vi "Model Initial Values - Fast Get Model Data.vi"(8 "error in (no error)":errorcluster, 11 "Local Model Ref in":T1 format="%.0x") -> (0 "error out":errorcluster, 1 "Inport Default Values":dbl[](array[numeric]), 2 "Inport Names":string[](array[string]), 3 "Local Model Ref out":T1 format="%.0x", 4 "Num Inports":i32, 5 "Inport Refs":T1[](array[typedef]) format="%.0x")   [LabVIEW 2011, in "Model Initial Values Custom Device.lvlib"]
uses:
  Model Initial Values Custom Device.lvlib
  <vilib>/NI Veristand/Custom Device API/Custom Device Item Ref.ctl
  Model Initial Values - Global.vi
  <vilib>/NI Veristand/Custom Device API/Get Item Property (Dependent Node Pointer).vi
  <vilib>/NI Veristand/Custom Device API/Get Item Property (String).vi
  <vilib>/NI Veristand/Custom Device API/Set Item Property (String).vi
  <vilib>/NI Veristand/Custom Device API/Set Item Property (String Array).vi
  <vilib>/NI Veristand/Custom Device API/Set Item Property (Double Array).vi
  <vilib>/NI Veristand/Custom Device API/Set Item Property (I32).vi
  <vilib>/NI Veristand/Custom Device API/Get Item Property (String Array).vi
  <vilib>/NI Veristand/Custom Device API/Get Item Property (Double Array).vi
  <vilib>/NI Veristand/Custom Device API/Get Item Property (I32).vi
  <vilib>/NI Veristand/Custom Device API/Custom Device API.lvlib
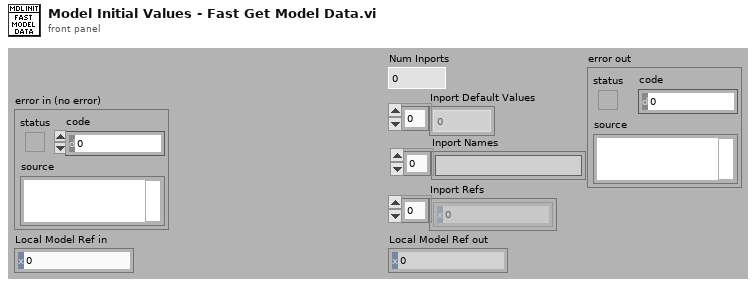
[diagram p1: front panel]
types:
  T1 = typedef "Custom Device API.lvlib/Custom Device Item Ref.ctl" = u64
  T2 = cluster{"Name":string, "Is Channel":bool, "GUID":string}
  T3 = cluster{"DLLSize":i32, "Timestamp":dbl, "MD5":string}
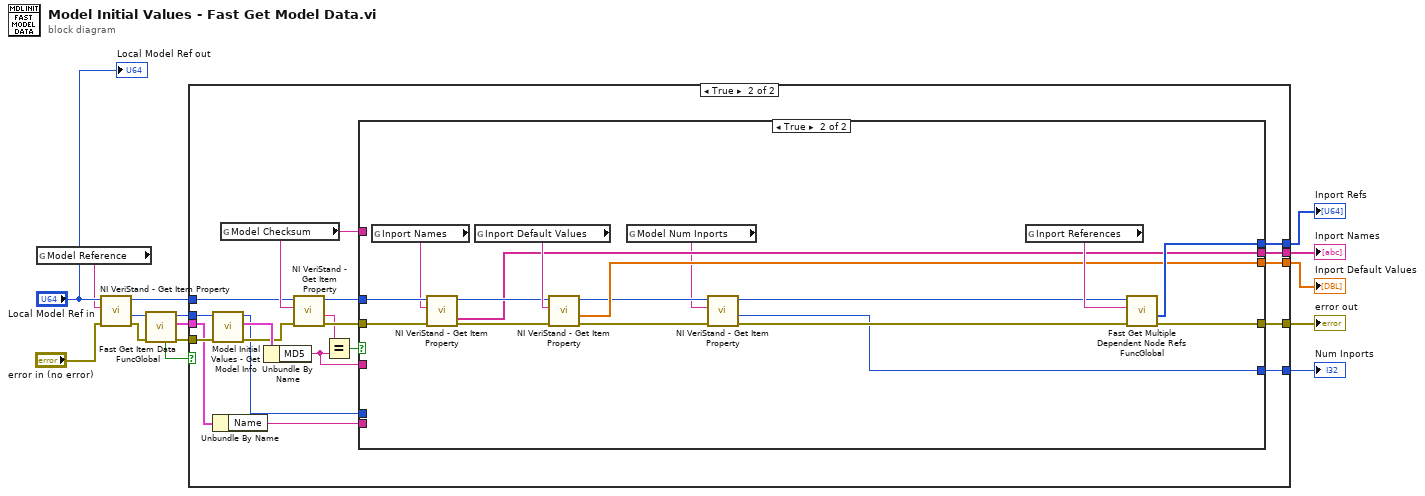
[diagram p0: block diagram]
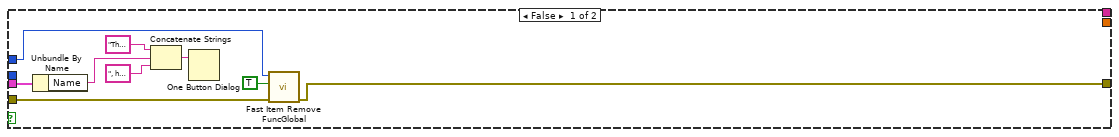
[diagram p2: hidden frame]
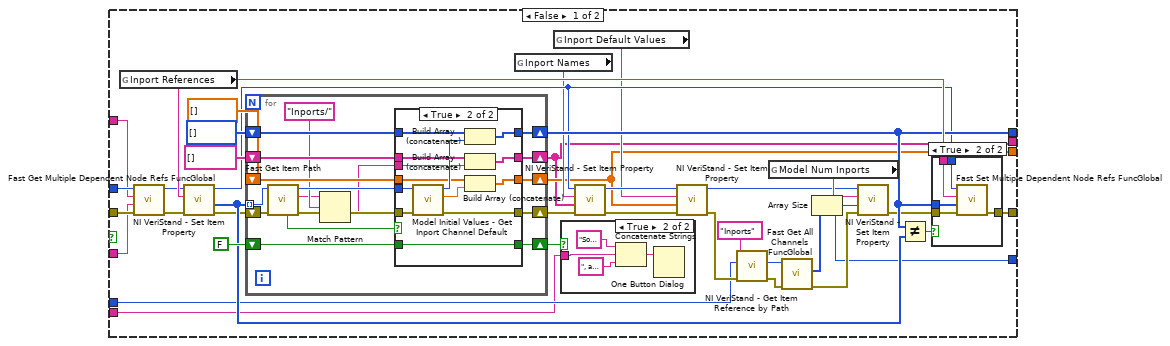
[diagram p3: hidden frame]
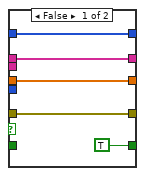
[diagram p6: hidden frame]
diagram:
  n1 = global read "Model Initial Values - Global.vi" "Model Reference"() -> (w12:string)
  n2 = call-poly <vilib>:"NI VeriStand - Get Item Property.vi"("error in (no error)"="error in (no error)", "Property Name"=w12, "Item Ref in"="Local Model Ref in") -> ("error out"=w6:errorcluster, "Dependent Node Ref"=w4:T1, "Item Ref out"=w14:T1)  [unwired: 5 in, 1 out]
  n3 = call "Fast Get Item Data FuncGlobal.vi"("error in (no error)"=w6, "Item Ref in"=w4) -> ("error out"=w5:errorcluster, "Item Info"=w2:T2, "Item Ref out"=w3:T1, "Found"=w1:bool)  [unwired: 6 in]
  n4 = case shown="True" w1 {
    tunnel: w14 -> [w17 w35]
    tunnel: [_ w33] -> w11
    tunnel: [_ w32] -> w10
    tunnel: [_ w31] -> w9
    tunnel: [_ w30] -> w8
    tunnel: [w16 w29] -> w7
    tunnel: w5 -> [w18 w28]
    tunnel: w3 -> [_ w27]
    tunnel: w2 -> [w24 w26]
    frame False {
      n5 = Unbundle By Name(w24) -> ("Name"=w19:string)
      n6 = Concatenate Strings("The model, " ("message"), w19, ", has been deleted from the project and will therefore be removed from this custom device." ("message")) -> (w22:string)
      n7 = One Button Dialog(message=w22) -> ()  [unwired: 1 in, 1 out]
      n8 = call "Fast Item Remove FuncGlobal.vi"("error in (no error)"=w18, "Force Delete (F)"=TRUE, "Item Ref in"=w17) -> ("error out"=w16:errorcluster)  [unwired: 7 in, 1 out]
    }
    frame True {
      n9 = call "Model Initial Values - Get Model Info.vi"("error in (no error)"=w28, "ID in"=w27) -> ("error out"=w42:errorcluster, "output cluster"=w43:T3, "ID out"=w34:T1)  [unwired: 7 in]
      n10 = Unbundle By Name(w26) -> ("Name"=w25:string)
      n11 = global read "Model Initial Values - Global.vi" "Model Checksum"() -> (w37:string)
      n12 = Unbundle By Name(w43) -> ("MD5"=w36:string)
      n13 = call-poly <vilib>:"NI VeriStand - Get Item Property.vi"("error in (no error)"=w42, "Property Name"=w37, "Item Ref in"=w35) -> ("error out"=w40:errorcluster, "Value"=w39:string, "Item Ref out"=w41:T1)  [unwired: 5 in, 1 out]
      n14 = Equal?(x=w39, y=w36) -> (x = y?=w38:bool)
      n15 = case shown="True" w38 {
        tunnel: [w76 w136] -> w29
        tunnel: w41 -> [w60 w141]
        tunnel: [w72 w134] -> w30
        tunnel: w40 -> [w63 w142]
        tunnel: w37 -> [w59 _]
        tunnel: w36 -> [w58 _]
        tunnel: [w57 w132] -> w32
        tunnel: [w56 w133] -> w31
        tunnel: [w45 w126] -> w33
        tunnel: w34 -> [w54 _]
        tunnel: w25 -> [w44 _]
        frame False {
          n16 = global read "Model Initial Values - Global.vi" "Inport References"() -> (w74:string)
          n17 = call-poly <vilib>:"NI VeriStand - Set Item Property.vi"("error in (no error)"=w63, "Value"=w58, "Property Name"=w59, "Item Ref in"=w60) -> ("error out"=w62:errorcluster, "Item Ref out"=w61:T1)  [unwired: 5 in, 1 out]
          n18 = call "Fast Get Multiple Dependent Node Refs FuncGlobal.vi"("error in (no error)"=w62, "Base Property Name"=w74, "Item Ref in"=w61) -> ("error out"=w71:errorcluster, "Dependent Node Refs"=w73:T1[], "Item Ref out"=w68:T1)  [unwired: 6 in]
          n19 = for {
            tunnel: w73 -> [w96] mode=indexing
            shift-right: [w106] -> w69
            shift-left: w71 -> [w100]
            shift-right: [w107] -> w56
            shift-left: string[] [] -> [w105]
            shift-right: [w103] -> w72
            shift-left: T1[] [] -> [w104]
            shift-right: [w102] -> w77
            shift-left: FALSE -> [w101]
            shift-right: [w94] -> w57
            shift-left: dbl[] [] -> [w95]
            n20 = call "Fast Get Item Path.vi"("error in (no error)"=w100, "Item Ref in"=w96) -> ("error out"=w99:errorcluster, "Path"=w92:string, "Item Ref out"=w97:T1, "Found"=w98:bool)  [unwired: 6 in]
            n21 = Match Pattern(string=w92, regular expression="Inports/") -> (after substring=w91:string)  [unwired: 1 in, 3 out]
            n22 = case shown="True" w98 {
              tunnel: [w111 w122] -> w107
              tunnel: w91 -> [_ w116]
              tunnel: w97 -> [_ w125]
              tunnel: w99 -> [w110 w124]
              tunnel: [w110 w123] -> w106
              tunnel: w105 -> [w111 w121]
              tunnel: w104 -> [w112 w119]
              tunnel: [w112 w118] -> w103
              tunnel: [TRUE w117] -> w102
              tunnel: w101 -> [_ w117]
              tunnel: w95 -> [w108 w114]
              tunnel: [w108 w113] -> w94
              frame False {
              }
              frame True {
                n23 = call "Model Initial Values - Get Inport Channel Default.vi"("error in"=w124, "Item Ref in"=w125) -> ("error out"=w123:errorcluster, "Default Value"=w115:dbl, "Item Ref out"=w120:T1)  [unwired: 6 in]
                n24 = Build Array (concatenate)(w119, w120) -> (w118:T1[])
                n25 = Build Array (concatenate)(w121, w116) -> (w122:string[])
                n26 = Build Array (concatenate)(w114, w115) -> (w113:dbl[])
              }
            }
          }
          n27 = global read "Model Initial Values - Global.vi" "Inport Names"() -> (w67:string)
          n28 = global read "Model Initial Values - Global.vi" "Inport Default Values"() -> (w64:string)
          n29 = case shown="True" w77 {
            tunnel: w44 -> [_ w87]
            frame False {
            }
            frame True {
              n30 = Concatenate Strings("Some inports have been deleted from the model, " ("message"), w87, ", and will therefore be removed from the \"Model Initial Values\" custom device." ("message")) -> (w88:string)
              n31 = One Button Dialog(message=w88) -> ()  [unwired: 1 in, 1 out]
            }
          }
          n32 = call-poly <vilib>:"NI VeriStand - Set Item Property.vi"("error in (no error)"=w69, "Value"=w56, "Property Name"=w67, "Item Ref in"=w68) -> ("error out"=w66:errorcluster, "Item Ref out"=w65:T1)  [unwired: 5 in, 1 out]
          n33 = call-poly <vilib>:"NI VeriStand - Set Item Property.vi"("error in (no error)"=w66, "Value"=w57, "Property Name"=w64, "Item Ref in"=w65) -> ("error out"=w55:errorcluster, "Item Ref out"=w46:T1)  [unwired: 5 in, 1 out]
          n34 = call <vilib>:"NI VeriStand - Get Item Reference by Path.vi"("error in (no error)"=w55, "Root Ref"=w54, "Item Path in"="Inports") -> ("error out"=w51:errorcluster, "Item Ref"=w52:T1)  [unwired: 5 in, 2 out]
          n35 = global read "Model Initial Values - Global.vi" "Model Num Inports"() -> (w49:string)
          n36 = call "Fast Get All Channels FuncGlobal.vi"("error in"=w51, "Section Ref in"=w52) -> ("error out"=w48:errorcluster, "Channel Refs"=w50:T1[])  [unwired: 6 in, 2 out]
          n37 = Array Size(array=w50) -> (size(s)=w45:i32)
          n38 = call-poly <vilib>:"NI VeriStand - Set Item Property.vi"("error in (no error)"=w48, "Value"=w45, "Property Name"=w49, "Item Ref in"=w46) -> ("error out"=w47:errorcluster)  [unwired: 5 in, 2 out]
          n39 = Not Equal?(x=w72, y=w73) -> (x != y?=w75:bool)
          n40 = case shown="True" w75 {
            tunnel: w68 -> [_ w83]
            tunnel: [w81 w84] -> w76
            tunnel: w74 -> [_ w85]
            tunnel: w72 -> [_ w86]
            tunnel: w47 -> [w81 w82]
            frame False {
            }
            frame True {
              n41 = call "Fast Set Multiple Dependent Node Refs FuncGlobal.vi"("error in (no error)"=w82, "Dependent Node Refs"=w86, "Base Property Name"=w85, "Item Ref in"=w83) -> ("error out"=w84:errorcluster)  [unwired: 6 in, 1 out]
            }
          }
        }
        frame True {
          n42 = global read "Model Initial Values - Global.vi" "Inport Names"() -> (w140:string)
          n43 = call-poly <vilib>:"NI VeriStand - Get Item Property.vi"("error in (no error)"=w142, "Property Name"=w140, "Item Ref in"=w141) -> ("error out"=w139:errorcluster, "Value"=w133:string[], "Item Ref out"=w137:T1)  [unwired: 5 in, 1 out]
          n44 = global read "Model Initial Values - Global.vi" "Inport Default Values"() -> (w138:string)
          n45 = call-poly <vilib>:"NI VeriStand - Get Item Property.vi"("error in (no error)"=w139, "Property Name"=w138, "Item Ref in"=w137) -> ("error out"=w131:errorcluster, "Value"=w132:dbl[], "Item Ref out"=w130:T1)  [unwired: 5 in, 1 out]
          n46 = global read "Model Initial Values - Global.vi" "Model Num Inports"() -> (w129:string)
          n47 = call-poly <vilib>:"NI VeriStand - Get Item Property.vi"("error in (no error)"=w131, "Property Name"=w129, "Item Ref in"=w130) -> ("error out"=w128:errorcluster, "Value"=w126:i32, "Item Ref out"=w127:T1)  [unwired: 5 in, 1 out]
          n48 = global read "Model Initial Values - Global.vi" "Inport References"() -> (w135:string)
          n49 = call "Fast Get Multiple Dependent Node Refs FuncGlobal.vi"("error in (no error)"=w128, "Base Property Name"=w135, "Item Ref in"=w127) -> ("error out"=w136:errorcluster, "Dependent Node Refs"=w134:T1[])  [unwired: 6 in, 1 out]
        }
      }
    }
  }
  "Num Inports" <- w11
  "Inport Default Values" <- w10
  "Inport Names" <- w9
  "Inport Refs" <- w8
  "error out" <- w7
  "Local Model Ref out" <- "Local Model Ref in"
